vi "GOLPI simple testing.vi"() -> ()   [LabVIEW 2013, in "GOLPI library.lvlib"]
uses:
  GOLPI library.lvlib
  Get Variable - polymorph parts/Get String.vi
  Get Variable - polymorph parts/Get Double.vi
  Get Variable - polymorph parts/Get Double Complex.vi
  Get Variable - polymorph parts/Get 1D Array Double.vi
  Get Variable - polymorph parts/Get 1D Array String.vi
  Get Variable - polymorph parts/Get 1D Array Double Complex.vi
  Get Variable - polymorph parts/Get 2D Array Double.vi
  Get Variable - polymorph parts/Get 2D Array Double Complex.vi
panel:
  in  "Bitstream":bool
  in  "hide debug console":bool
  in  "data type array 5":cdb[][](array[numeric])
  in  "data type array 4":dbl[][](array[numeric])
  in  "use temporary file?":bool
  in  "data type array 3":cdb[](array[numeric])
  in  "data type array 2":string[](array[string])
  in  "data type 4":cdb
  in  "data type 3":dbl
  in  "Get variable":T1(tab)=enum."vector reals"
  out "s":string
  out "r":dbl format="%.2f"
  out "c":cdb format="%.2f"
  out "vs length":i32
  out "vs":string[](array[string])
  out "vr":dbl[](array[numeric])
  out "vr length":i32
  out "vc length":i32
  out "vc":cdb[](array[numeric])
  out "mr":dbl[][](array[numeric]) format="%.2f"
  out "mr sizes":i32[](array[numeric])
  out "mc sizes":i32[](array[numeric])
  out "mc":cdb[][](array[numeric]) format="%.2f"
  in  "data type array":dbl[](array[numeric])
  in  "data type":string
  in  "variable name":string="x"
  in  "command":string="x=[1 2 3]\ndisp('OK')"
  out "GNU Octave version":string
  out "exit code":i32
  out "error out":errorcluster
  out "read buffer":string
  in  "Octave binary directory":path=path "C:/Program Files/Octave-3.6.2/bin"
  in  "Working directory":path=path "C:/"
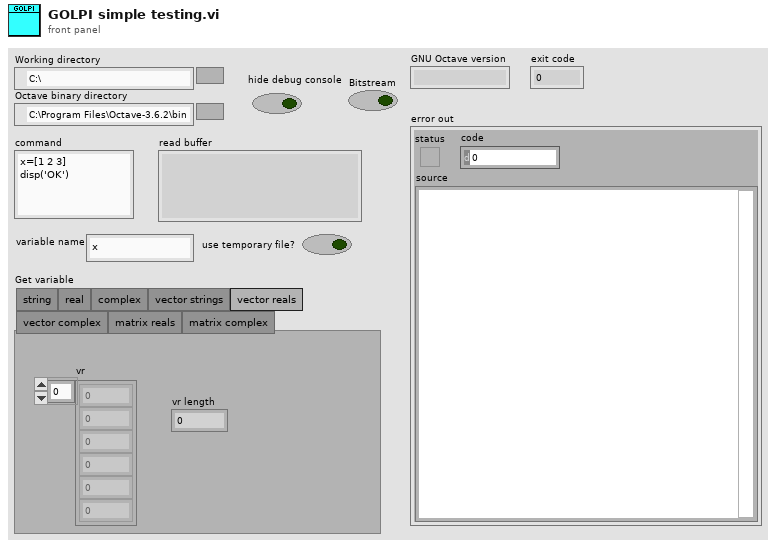
[diagram p1: front panel]
types:
  T1 = enum32{"string", "real", "complex", "vector strings", "vector reals", "vector complex", "matrix reals", "matrix complex"}
  T2 = typedef "GOLPI library.lvlib/GOLPI reference Type Def.ctl" = cluster{"pipe handle":T3, "fast read timeout [ms]":u32, "fast read settle time [ms]":u32, "fast read to multiple [ms]":u32, "max elements per input line":u32, "slow read timeout [ms]":u32, "stdin double format specifier":string, "max elements per stdout output column":u32, "console mode bitstream":bool, "bitstream first read timeout [ms]":u32, "bitstream read timeout [ms]":u32}
  T3 = typedef "LV Process library.lvlib/Pipe Handle.ctl" = cluster{"lv_proc.dll file path":path, "process instance handle":u32[], "debug mode":bool, "debug data":cluster{"time":timestamp, "stdin":bool, "data":string}[]}
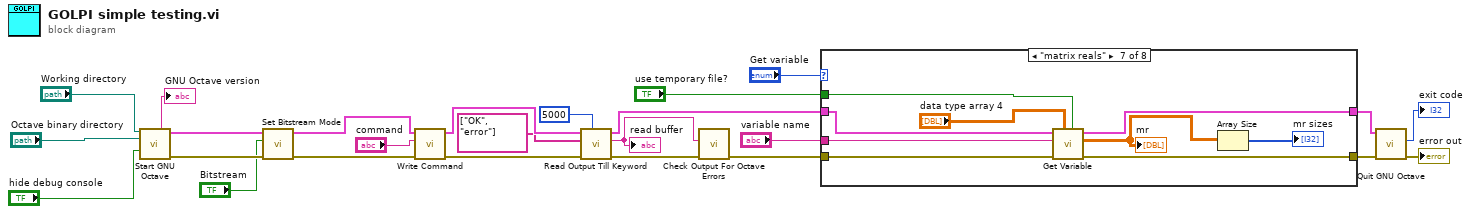
[diagram p0: block diagram]
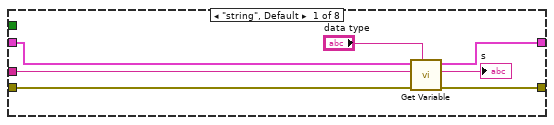
[diagram p2: hidden frame]
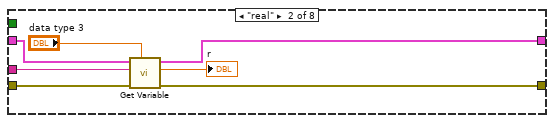
[diagram p3: hidden frame]
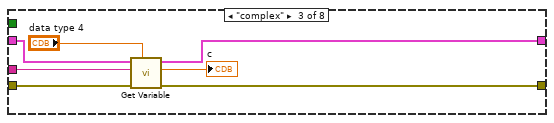
[diagram p4: hidden frame]
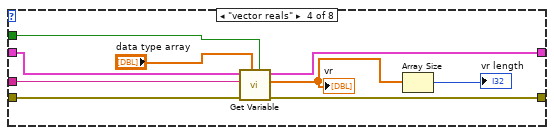
[diagram p5: hidden frame]
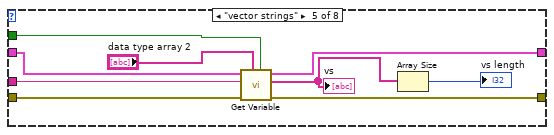
[diagram p6: hidden frame]
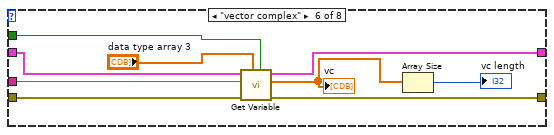
[diagram p7: hidden frame]
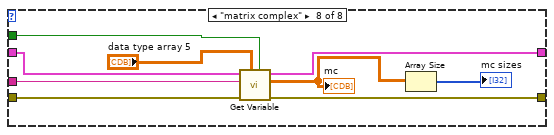
[diagram p8: hidden frame]
diagram:
  n1 = call "Start GNU Octave.vi"("working directory"="Working directory", "octave exe file or directory"="Octave binary directory", "hide debug console (T)"="hide debug console") -> ("GNU Octave version"=→"GNU Octave version":string, "GOLPI ref. out"=w3:T2, "error out"=w5:errorcluster)  [unwired: 9 in, 1 out]
  n2 = call "Set Bitstream Mode.vi"("error in"=w5, "Bitstream mode (F)"="Bitstream", "GOLPI ref. in"=w3) -> ("error out"=w4:errorcluster, "GOLPI ref. out"=w2:T2)  [unwired: 7 in]
  n3 = call "Write Command.vi"("error in"=w4, "command"="command", "GOLPI ref. in"=w2) -> ("error out"=w22:errorcluster, "GOLPI ref. out"=w23:T2)  [unwired: 7 in]
  n4 = call "Read Output Till Keyword.vi"("timeout [ms]"=u32 5000, "error in"=w22, "keywords"=string[] ["OK", "error"], "GOLPI ref. in"=w23) -> ("error out"=w15:errorcluster, "read buffer"=w13:string, "GOLPI ref. out"=w19:T2)  [unwired: 4 in, 1 out]
  "read buffer" <- w13
  n5 = call "Check Output For Octave Errors.vi"("error in"=w15, "read buffer"=w13) -> ("error out"=w14:errorcluster)  [unwired: 9 in]
  n6 = case shown="\"matrix reals\"" "Get variable" {
    tunnel: w19 -> [w31 w36 w44 w53 w61 w69 w82 w90]
    tunnel: [w28 w34 w41 w52 w58 w66 w78 w87] -> w18
    tunnel: [w29 w33 w40 w51 w59 w67 w79 w86] -> w17
    tunnel: "variable name" -> [w26 w37 w42 w54 w62 w70 w81 w88]
    tunnel: w14 -> [w30 w38 w43 w55 w60 w68 w80 w89]
    tunnel: "use temporary file?" -> [_ _ _ w48 w56 w65 w77 w85]
    frame "string", Default {
      n7 = call-poly "Get Variable.vi"("data type of variable"="data type", "error in"=w30, "variable name"=w26, "GOLPI ref. in"=w31) -> ("error out"=w29:errorcluster, "value"=→"s":string, "GOLPI ref. out"=w28:T2)  [unwired: 5 in]
    }
    frame "real" {
      n8 = call-poly "Get Variable.vi"("data type of variable"="data type 3", "error in"=w38, "variable name"=w37, "GOLPI ref. in"=w36) -> ("error out"=w33:errorcluster, "value"=→"r":dbl, "GOLPI ref. out"=w34:T2)  [unwired: 5 in]
    }
    frame "complex" {
      n9 = call-poly "Get Variable.vi"("data type of variable"="data type 4", "error in"=w43, "variable name"=w42, "GOLPI ref. in"=w44) -> ("error out"=w40:errorcluster, "value"=→"c":cdb, "GOLPI ref. out"=w41:T2)  [unwired: 5 in]
    }
    frame "vector reals" {
      n10 = call-poly "Get Variable.vi"("use temporary file? (F)"=w48, "data type of variable"="data type array", "error in"=w55, "variable name"=w54, "GOLPI ref. in"=w53) -> ("error out"=w51:errorcluster, "value"=w47:dbl[], "GOLPI ref. out"=w52:T2)  [unwired: 4 in]
      "vr" <- w47
      n11 = Array Size(array=w47) -> (size(s)=→"vr length":i32)
    }
    frame "vector strings" {
      n12 = call-poly "Get Variable.vi"("use temporary file? (F)"=w56, "data type of variable"="data type array 2", "error in"=w60, "variable name"=w62, "GOLPI ref. in"=w61) -> ("error out"=w59:errorcluster, "value"=w57:string[], "GOLPI ref. out"=w58:T2)  [unwired: 4 in]
      "vs" <- w57
      n13 = Array Size(array=w57) -> (size(s)=→"vs length":i32)
    }
    frame "vector complex" {
      n14 = call-poly "Get Variable.vi"("use temporary file? (F)"=w65, "data type of variable"="data type array 3", "error in"=w68, "variable name"=w70, "GOLPI ref. in"=w69) -> ("error out"=w67:errorcluster, "value"=w71:cdb[], "GOLPI ref. out"=w66:T2)  [unwired: 4 in]
      "vc" <- w71
      n15 = Array Size(array=w71) -> (size(s)=→"vc length":i32)
    }
    frame "matrix reals" {
      n16 = call-poly "Get Variable.vi"("use temporary file? (F)"=w77, "data type of variable"="data type array 4", "error in"=w80, "variable name"=w81, "GOLPI ref. in"=w82) -> ("error out"=w79:errorcluster, "value"=w74:dbl[][], "GOLPI ref. out"=w78:T2)  [unwired: 4 in]
      "mr" <- w74
      n17 = Array Size(array=w74) -> (size(s)=→"mr sizes":i32[])
    }
    frame "matrix complex" {
      n18 = call-poly "Get Variable.vi"("use temporary file? (F)"=w85, "data type of variable"="data type array 5", "error in"=w89, "variable name"=w88, "GOLPI ref. in"=w90) -> ("error out"=w86:errorcluster, "value"=w83:cdb[][], "GOLPI ref. out"=w87:T2)  [unwired: 4 in]
      "mc" <- w83
      n19 = Array Size(array=w83) -> (size(s)=→"mc sizes":i32[])
    }
  }
  n20 = call "Quit GNU Octave.vi"("error in"=w17, "GOLPI ref. in"=w18) -> ("error out"=→"error out":errorcluster, "exit code"=→"exit code":i32)  [unwired: 8 in]
